vi "Send dpo config.vi"(0 "Array Configuration":string[](array[string]), 1 "TCP/IP Addres":string) -> (2 "error out":errorcluster, 3 "Boolean":bool, 4 "Exit":bool)   [LabVIEW 2010]
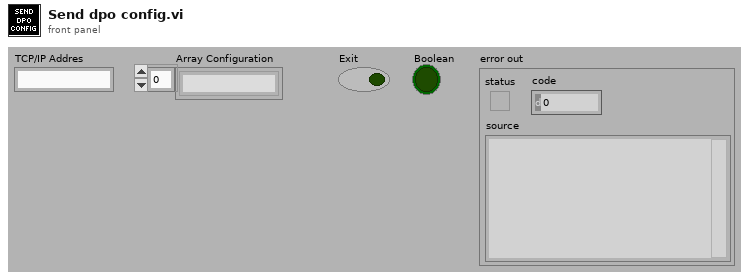
[diagram p1: front panel]
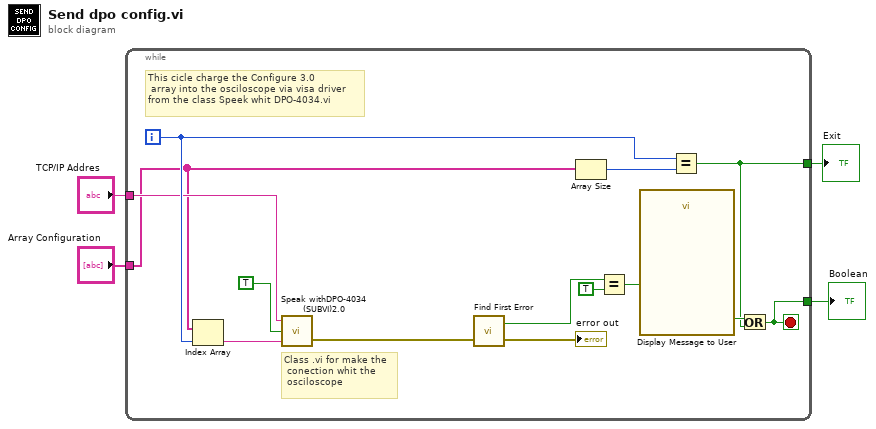
[diagram p0: block diagram]
diagram:
  n1 = while {
    tunnel: "TCP/IP Addres" -> [w9]
    tunnel: [w7] -> w1
    tunnel: "Array Configuration" -> [w6]
    tunnel: [w5] -> w4
    i -> [w17]
    stop <- w5 stop-if-true
    # "Class .vi for make the\n conection whit the\n osciloscope"
    # "This cicle charge the Configure 3.0\n array into the osciloscope via visa driver \nfrom the class Speek whit DPO-4034.vi"
    n2 = Index Array "Index Array"(array=w6, index=w17) -> (element=w18:string)
    n3 = call "Speak withDPO-4034 (SUBVI)2.0.vi"("Send Command"=w18, "Send:  TRUE\nRecive: FALSE"=TRUE, "VISA Resource Name"=w9) -> ("error out"=w14:errorcluster)  [unwired: 1 out]
    n4 = call <vilib>:"Find First Error.vi"("error in (no error)"=w14) -> ("error out"=→"error out":errorcluster, "error?"=w10:bool)  [unwired: 3 in]
    n5 = Array Size(array=w6) -> (size(s)=w16:i32)
    n6 = Equal?(x=w10, y=TRUE) -> (x = y?=w12:bool)
    n7 = call "Display Message to User"("Enable"=w12) -> ("OK"=w8:bool)  [unwired: 9 in, 1 out]
    n8 = Equal?(x=w17, y=w16) -> (x = y?=w7:bool)
    n9 = Or(x=w8, y=w7) -> (x .or. y?=w5:bool)
  }
  "Exit" <- w1
  "Boolean" <- w4
